vi "Read Attributes.vi"(11 "Close Application Msg":refnum<class "Close Application Msg.lvclass">) -> (2 "Payload":cluster{"Close Application":bool})   [LabVIEW 2017, in "User Interface.lvlib" / "Close Application Msg.lvclass"]
uses:
  Close Application Msg.lvclass
  Close Application Msg.lvclass/Close Application Msg.ctl
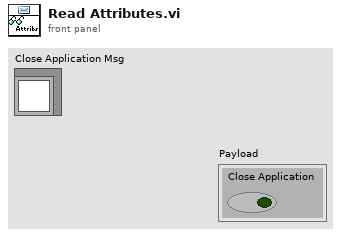
[diagram p1: front panel]
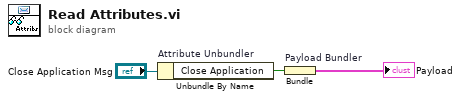
[diagram p0: block diagram]
diagram:
  n1 = Unbundle By Name "Attribute Unbundler"("Close Application Msg") -> ("Close Application"=w1:bool)
  n2 = Bundle "Payload Bundler"("Close Application"=w1) -> (→"Payload":cluster{"Close Application":bool})  [unwired: 1 in]
